vi "SetScanFuncTree.vi"(8 "error in (no error)":errorcluster caption="entrée d'erreur (pas d'erreur)", 10 "ScanTreeRef":refnum<vi>, 11 "Experiment en entrée":refnum<class "Experiment.lvclass"> caption="DNL_LabVIEW Object in") -> (0 "error out":errorcluster caption="sortie d'erreur", 3 "Experiment en sortie":refnum<class "Experiment.lvclass"> caption="DNL_LabVIEW Object out")   [LabVIEW 2019, in "Experiment.lvclass"]
uses:
  Experiment.lvclass
  Experiment.lvclass/Experiment.ctl
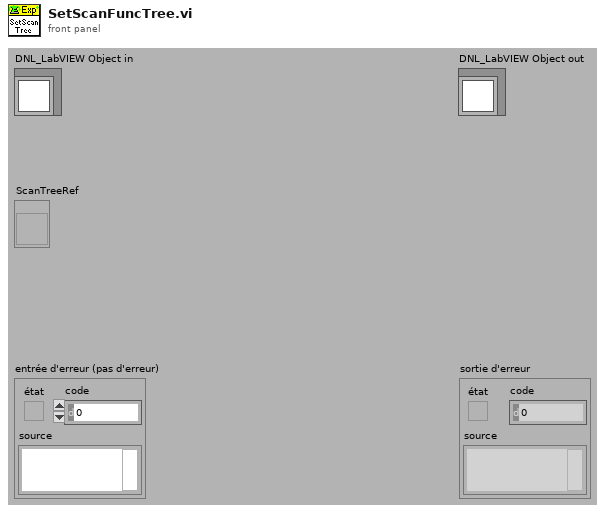
[diagram p1: front panel]
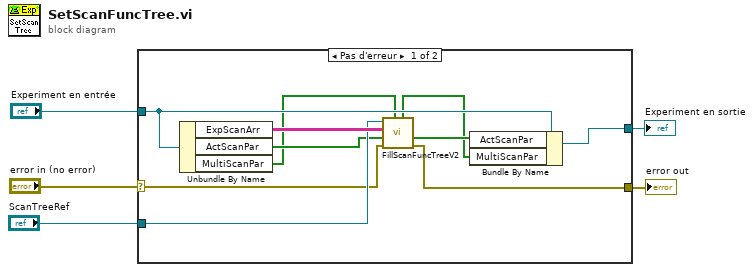
[diagram p0: block diagram]
diagram:
  n1 = case shown="Pas d'erreur" "error in (no error)" {
    selector: "error in (no error)" -> [w9 w17]
    tunnel: [w8 w17] -> w4
    tunnel: [w10 w16] -> w2
    tunnel: "Experiment en entrée" -> [w11 w16]
    tunnel: "ScanTreeRef" -> [w14 _]
    frame No Error {
      n2 = Unbundle By Name(w11) -> ("ExpScanArr"=w15:string[][], "ActScanPar"=w13:bool[], "MultiScanPar"=w7:bool[])
      n3 = call "FillScanFuncTreeV2.vi"("Multi ScanPar"=w7, "ErrorIn(No Error)"=w9, "Active ScanPar"=w13, "ScanFunc"=w15, "ScanTreeRef"=w14) -> ("sortie d'erreur"=w8:errorcluster, "Active ScanParOut"=w12:bool[], "Multi ScanParOut"=w6:bool[])  [unwired: 4 in]
      n4 = Bundle By Name(cluster=w11, "ActScanPar"=w12, "MultiScanPar"=w6) -> (w10:refnum<class "Experiment.lvclass">)
    }
    frame Error {
    }
  }
  "error out" <- w4
  "Experiment en sortie" <- w2
